vi "Name Value Read Tags.vi"(0 "Path":path, 11 "Error In":errorcluster) -> (4 "Group Names":string[](array[string]), 6 "Tags":string[][][](array[string]), 8 "Notes":string, 15 "Error Out":errorcluster)   [LabVIEW 2020]
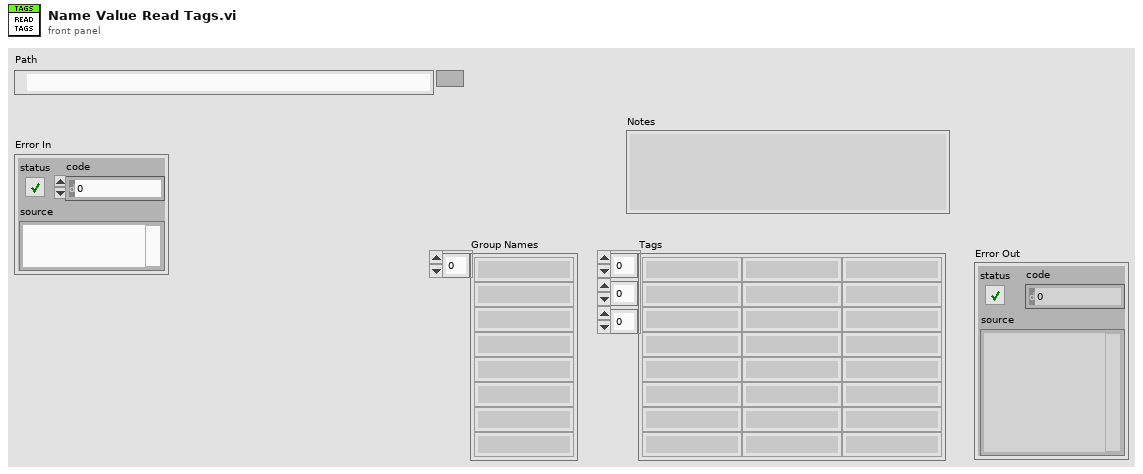
[diagram p1: front panel]
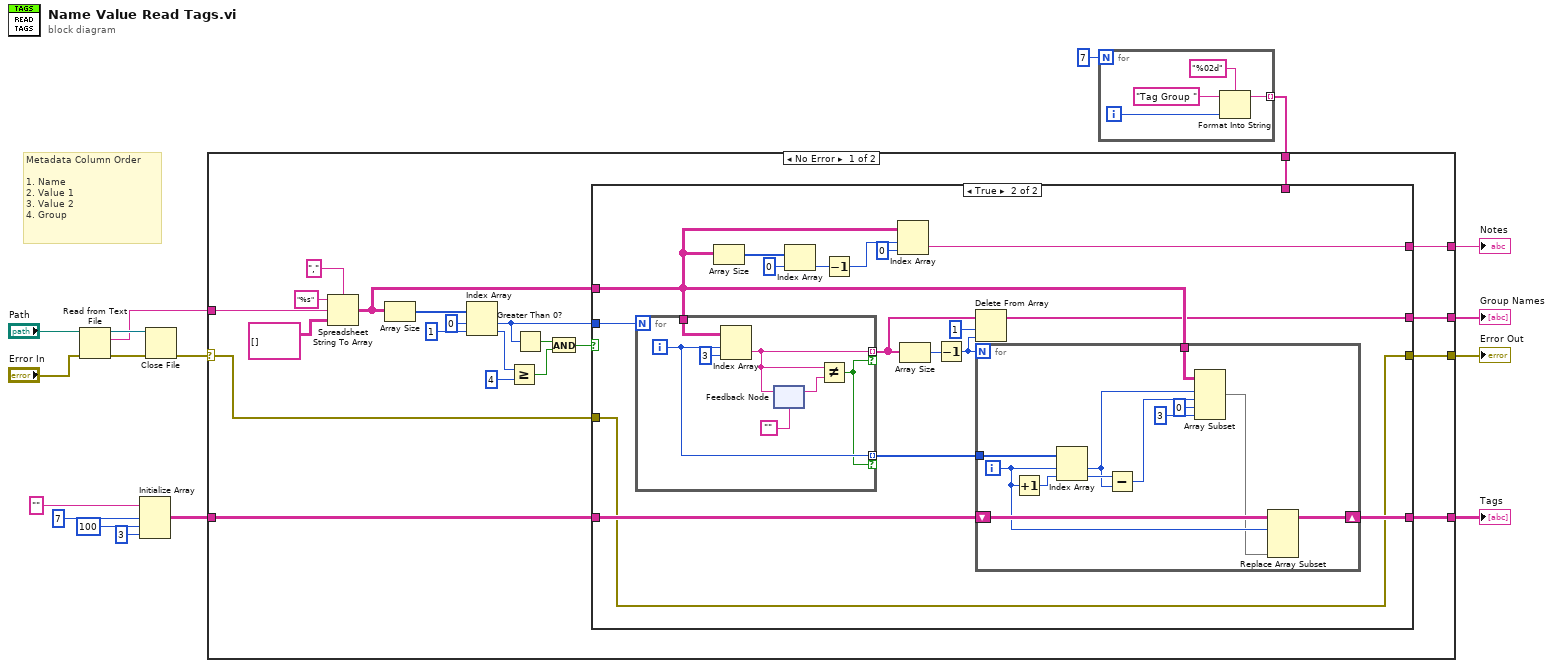
[diagram p0: block diagram]
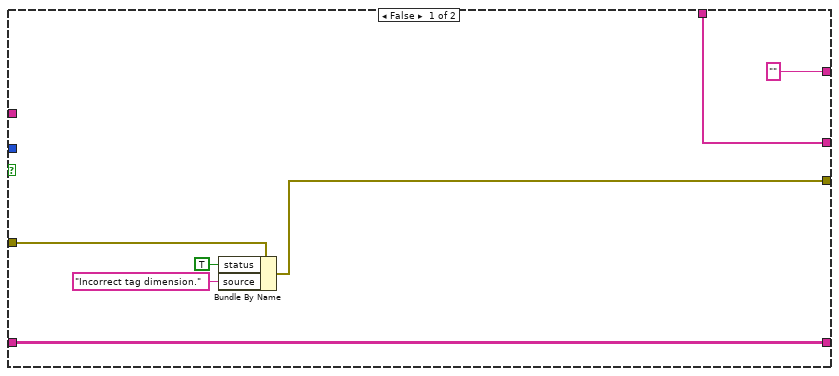
[diagram p2: hidden frame]
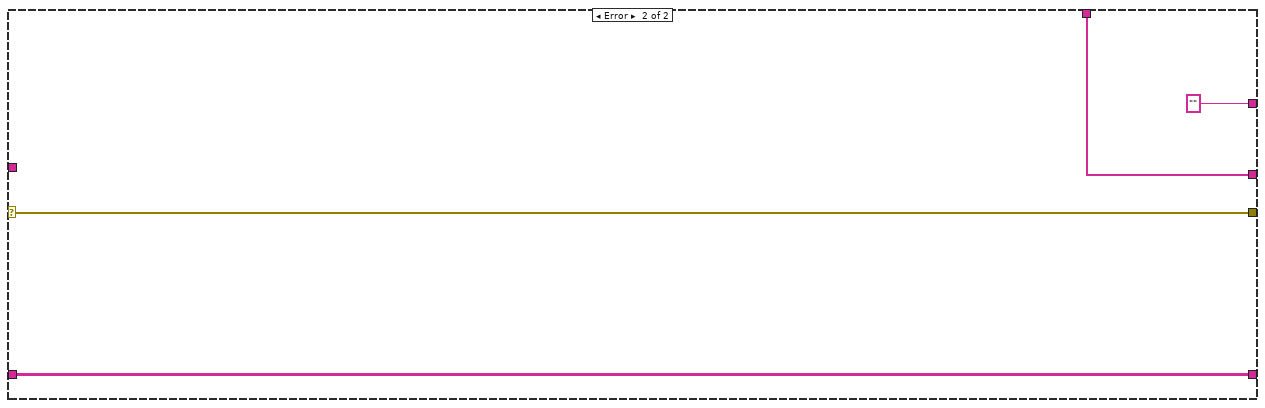
[diagram p3: hidden frame]
diagram:
  # "Metadata Column Order\n\n1. Name\n2. Value 1\n3. Value 2\n4. Group"
  n1 = Read from Text File(file (use dialog)="Path", error in="Error In") -> (refnum out=w16:refnum<file>, text=w12:string, error out=w14:errorcluster)  [unwired: 2 in, 1 out]
  n2 = Initialize Array("", 7 ("dimension size"), 100 ("dimension size"), 3 ("dimension size")) -> (w5:string[][][])
  n3 = Close File(refnum=w16, error in=w14) -> (error out=w13:errorcluster)  [unwired: 1 out]
  n4 = for {
    N: 7 -> [_]
    tunnel: [w18] -> w4 mode=indexing
    i -> [w19]
    n5 = Format Into String(format string="%02d", initial string="Tag Group ", w19) -> (resulting string=w18:string)  [unwired: 1 in, 1 out]
  }
  n6 = case shown="No Error" w13 {
    selector: w13 -> [w24 w89]
    tunnel: w12 -> [w42 _]
    tunnel: [w23 w89] -> w3
    tunnel: [w29 w86] -> w11
    tunnel: [w28 w88] -> w10
    tunnel: [w27 ""] -> w9
    tunnel: w5 -> [w26 w86]
    tunnel: w4 -> [w25 w88]
    frame No Error {
      n7 = Spreadsheet String To Array(delimiter (Tab)=",", format string="%s", spreadsheet string=w42, array type (2D Dbl)=string[][] []) -> (array=w30:string[][])
      n8 = Array Size(array=w30) -> (size(s)=w39:i32[])
      n9 = Index Array(array=w39, index #1=0 ("index"), index #2=1 ("index")) -> (element #1=w31:i32, element #2=w35:i32)
      n10 = Greater Or Equal?(x=w35, y=4) -> (x >= y?=w33:bool)
      n11 = Greater Than 0?(x=w31) -> (x > 0?=w36:bool)
      n12 = And(x=w36, y=w33) -> (x .and. y?=w32:bool)
      n13 = case shown="True" w32 {
        tunnel: w31 -> [_ w66]
        tunnel: w30 -> [_ w59]
        tunnel: w26 -> [w48 w63]
        tunnel: [w48 w62] -> w29
        tunnel: [w47 w53] -> w28
        tunnel: ["" w56] -> w27
        tunnel: w25 -> [w47 _]
        tunnel: w24 -> [w46 w50]
        tunnel: [w44 w50] -> w23
        frame False {
          n14 = Bundle By Name(cluster=w46, "status"=TRUE, "source"="Incorrect tag dimension.") -> (w44:errorcluster)
        }
        frame True {
          n15 = for {
            N: w66 -> [_]
            tunnel: [w82] -> w64 mode=indexing if=w80
            tunnel: [w81] -> w54 mode=indexing if=w80
            tunnel: w59 -> [w79]
            i -> [w82]
            n16 = Index Array(array=w79, index (row)=w82, index (col)=3 ("disabled index (col)")) -> (element=w81:string)
            n17 = feedback-in #1(w81) -> ()
            n18 = feedback #1("") -> (w84:string)
            n19 = Not Equal?(x=w81, y=w84) -> (x != y?=w80:bool)
          }
          n20 = Array Size(array=w59) -> (size(s)=w61:i32[])
          n21 = Index Array(array=w61, index=0) -> (element=w58:i32)
          n22 = Decrement(x=w58) -> (x-1=w55:i32)
          n23 = Index Array(array=w59, index (row)=w55, index (col)=0 ("disabled index (col)")) -> (element=w56:string)
          n24 = Array Size(array=w54) -> (size(s)=w65:i32)
          n25 = Decrement(x=w65) -> (x-1=w51:i32)
          n26 = Delete From Array(array=w54, length=1, index=w51) -> (array with subset deleted=w53:string[])  [unwired: 1 out]
          n27 = for {
            N: w51 -> [_]
            tunnel: w64 -> [w78]
            tunnel: w59 -> [w75]
            shift-right: [w69] -> w62
            shift-left: w63 -> [w70]
            i -> [w68]
            n28 = Increment(x=w68) -> (x+1=w77:i32)
            n29 = Index Array(array=w78, index #1=w68, index #2=w77) -> (element #1=w74:i32, element #2=w76:i32)
            n30 = Subtract(x=w76, y=w74) -> (x-y=w71:i32)
            n31 = Array Subset(array=w75, index (row)=w74, length (row)=w71, index (col)=0 ("index"), length (col)=3 ("length")) -> (w67:string[][])
            n32 = Replace Array Subset(array=w70, new element=w67, index (dim 0)=w68) -> (w69:string[][][])  [unwired: 2 in]
          }
        }
      }
    }
    frame Error {
    }
  }
  "Notes" <- w9
  "Group Names" <- w10
  "Tags" <- w11
  "Error Out" <- w3
